vi "Resize Panel to Pane.vi"(8 "error in (no error)":errorcluster, 10 "Apply Recursively? (F)":bool, 11 "IViewable In":refnum<class "IViewable.lvclass">) -> (0 "error out":errorcluster, 3 "IViewable Out":refnum<class "IViewable.lvclass">)   [LabVIEW 2020, in "IViewable.lvlib" / "IViewable.lvclass"]
doc: "抽象方法\n将面板调整为窗格"
uses:
  IViewable.lvclass
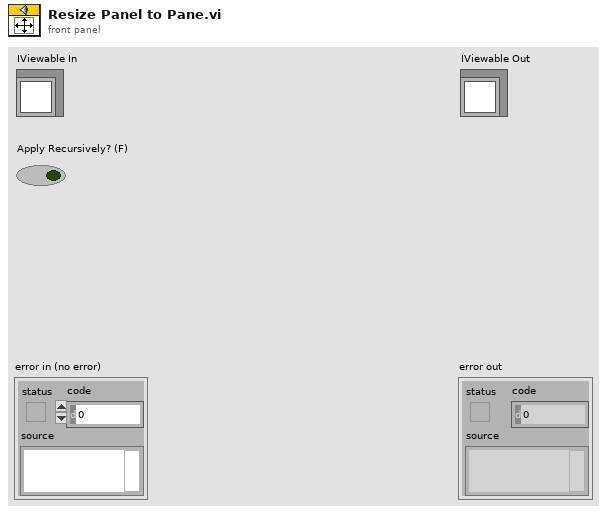
[diagram p1: front panel]
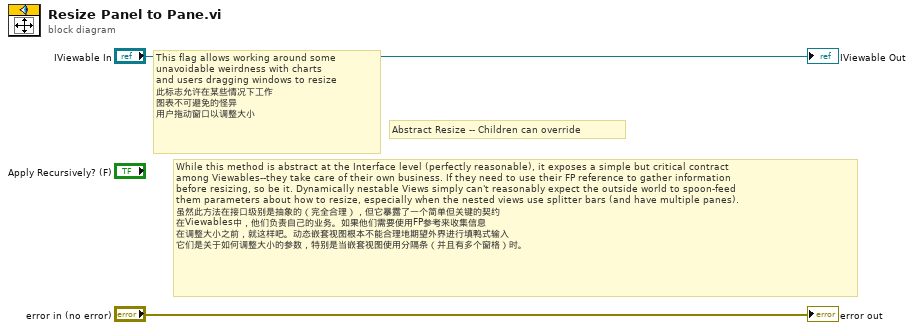
[diagram p0: block diagram]
diagram:
  # "This flag allows working around some\nunavoidable weirdness with charts\nand users dragging windows to resize\n此标志允许在某些情况下工作\n图表不可避免的怪异\n用户拖动窗口以调整大小"
  # "While this method is abstract at the Interface level (perfectly reasonable), it exposes a simple but critical contract\namong Viewables--they take care of their own business. If they need to use their FP reference to gather information\nbefore resizing, so be it. Dynamically nestable Views simply can't reasonably expect the outside world to spoon-feed\nthem parameters about how to resize, especially when the nested views use splitter bars (and have multiple panes).\n虽然此方法在接口级别是抽象的（完全合理），但它暴露了一个简单但关键的契约\n在Viewables中，他们负责自己的业务。如果他们需要使用FP参考来收集信息\n在调整大小之前，就这样吧。动态嵌套视图根本不能合理地期望外界进行填鸭式输入\n它们是关于如何调整大小的参数，特别是当嵌套视图使用分隔条（并且有多个窗格）时。"
  # "Abstract Resize -- Children can override"
  "error out" <- "error in (no error)"
  "IViewable Out" <- "IViewable In"
